vi "LAUNCHER.vi"   [LabVIEW 2019]
uses:
  C:/Program Files (x86)/National Instruments/LabVIEW 2019/vi.lib/ActorFramework/Actor/Actor.lvclass
  <vilib>/ActorFramework/Actor/Actor.lvclass
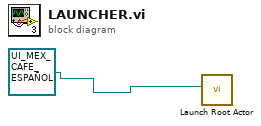
[diagram p0: block diagram]
diagram:
  n1 = call <vilib>:"Launch Root Actor.vi"("Actor"=refnum<class "UI_MEX_CAFE_ESPAÑOL.lvclass"> refnum ("UI_MEX_CAFE_ESPAÑOL.lvlib:UI_MEX_CAFE_ESPAÑOL.lvclass")) -> ()  [unwired: 9 in, 2 out]
